vi "Begin.vi"() -> (0 "Error Out":errorcluster)   [LabVIEW 2019]
doc: "Called before other user functions, this VI is expected to open initial I/O refnums, load in file data, and do all program initialization. Notice that the <B>error out</B> terminal is simply used for data flow. Wiring it to other structures or subVIs ensures that this VI runs first."
uses:
  dsdata.vi
  <vilib>/Rock Robotics/WPI/DriverStation/WPI_DriverStationRobotMode2.ctl
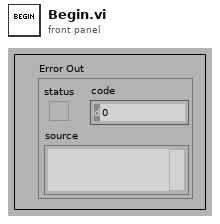
[diagram p1: front panel]
types:
  T1 = typedef "WPI_DriverStationRobotMode2.ctl" = enum16{"Autonomous Disabled", "Autonomous Enabled", "Teleop Disabled", "Teleop Enabled", "Disconnected", "Finish", "Test Disabled", "Test Enabled", "Emergency Stopped"}
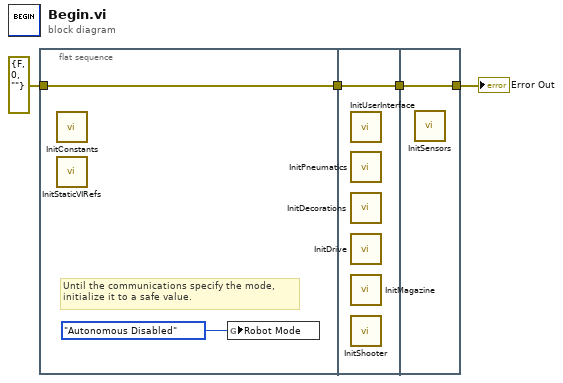
[diagram p0: block diagram]
diagram:
  n1 = flat-sequence {
    tunnel: [w6] -> w4
    tunnel: errorcluster {"status"=FALSE, "code"=0, "source"=""} ("error in") -> [w6]
    tunnel: w4 -> [w7]
    tunnel: [w7] -> w2
    tunnel: w2 -> [w8]
    tunnel: [w8] -> w1
    frame #0 {
      # "Until the communications specify the mode,\ninitialize it to a safe value."
      n2 = call "InitConstants.vi"() -> ()  [unwired: 12 in]
      n3 = call "InitStaticVIRefs.vi"() -> ()  [unwired: 12 in]
      n4 = global write "dsdata.vi" "Robot Mode"(WPI_DriverStationRobotMode2."Autonomous Disabled" ("Robot Mode")) -> ()
    }
    frame #1 {
      n5 = call "InitUserInterface.vi"() -> ()  [unwired: 12 in]
      n6 = call "InitPneumatics.vi"() -> ()  [unwired: 12 in]
      n7 = call "InitDecorations.vi"() -> ()  [unwired: 12 in]
      n8 = call "InitDrive.vi"() -> ()  [unwired: 1 in]
      n9 = call "InitMagazine.vi"() -> ()  [unwired: 1 in]
      n10 = call "InitShooter.vi"() -> ()  [unwired: 12 in]
    }
    frame #2 {
      n11 = call "InitSensors.vi"() -> ()  [unwired: 1 in]
    }
  }
  "Error Out" <- w1
